vi "134 - Pro - Con (Saved).vi"() -> ()   [LabVIEW 2020]
doc: "Use this template to build a producer/consumer design pattern. Use this template when you need to execute a process, such as data analysis, when a data source, such as a triggered acquisition, produces data at an uneven rate and you need to execute the process when the data becomes available."
uses:
  <vilib>/Utility/error.llb/DialogType.ctl
  <vilib>/DAQmx/read.llb/DAQmx Read (Analog Wfm 1Chan NSamp).vi
  <vilib>/DAQmx/create/channels.llb/DAQmx Create Channel (AI-Voltage-Basic).vi
  <vilib>/DAQmx/configure/timing.llb/DAQmx Timing (Sample Clock).vi
  <vilib>/Analysis/0measdsp.llb/Scaled Time Domain Window (DBL).vi
  <vilib>/DAQmx/miscellaneous.llb/DAQmx Fill In Error Info.vi
  <vilib>/Analysis/NI_AALPro.lvlib
panel:
  in  "Sample per Channel":dbl
  out "dt":dbl
  out "Frequency Peak":dbl format="%0.4f"
  in  "Filename":path=path "C:/Users/Hung/Desktop/TestSave.tdms"
  out "Record Signal":waveform(dbl)(graph)
  in  "Compare":dbl
  out "Filename Out":path
  in  "Saving":bool
  out "RMS":dbl
  out "Numeric 2":i32
  out "Numeric":i32
  out "Waveform Graph":waveform(dbl)(graph)
  out "Data (Consumer Loop)":dbl[](array[numeric])
  in  "stop":bool
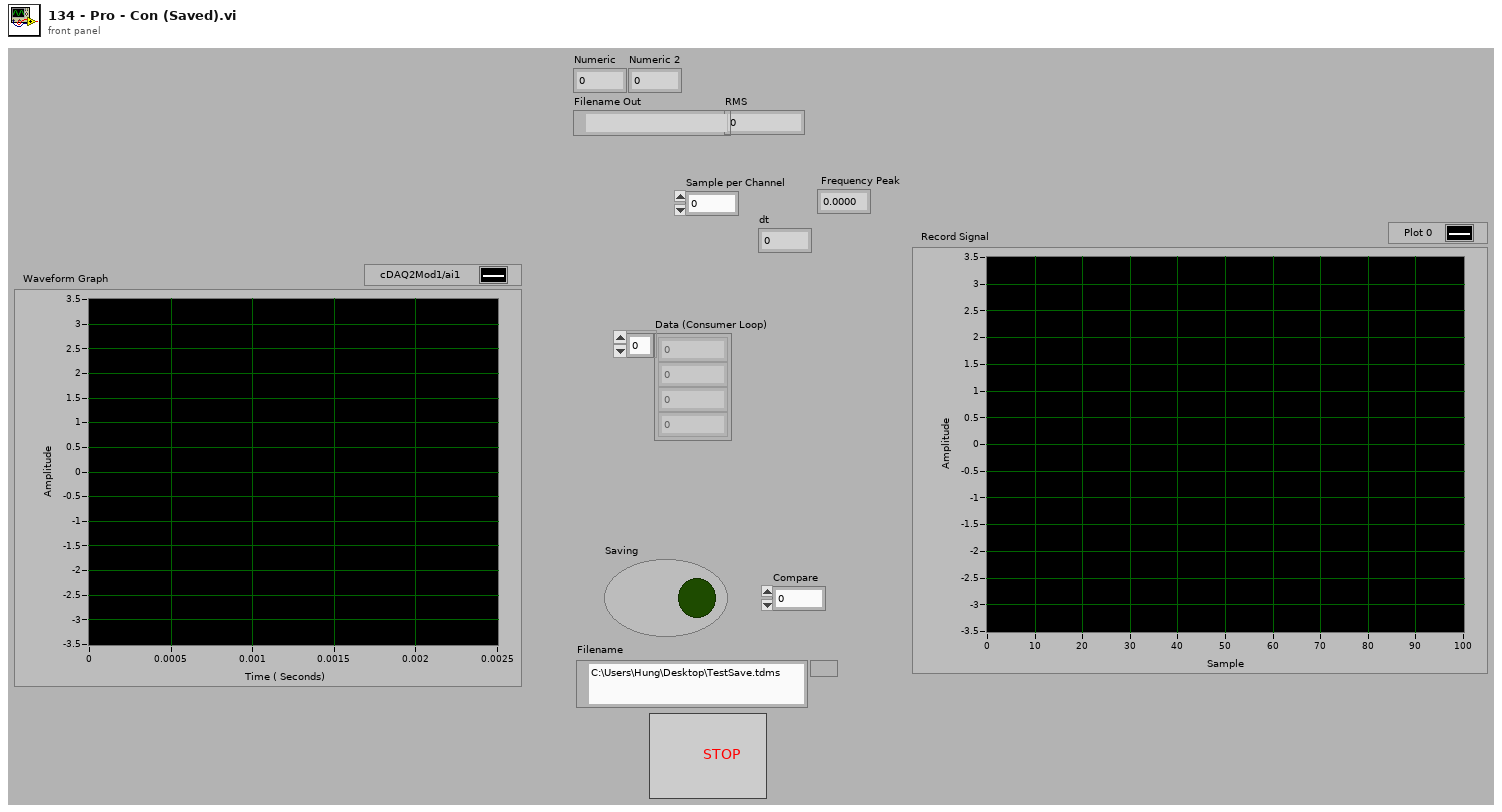
[diagram p1: front panel]
types:
  T1 = typedef "DialogType.ctl" = u16
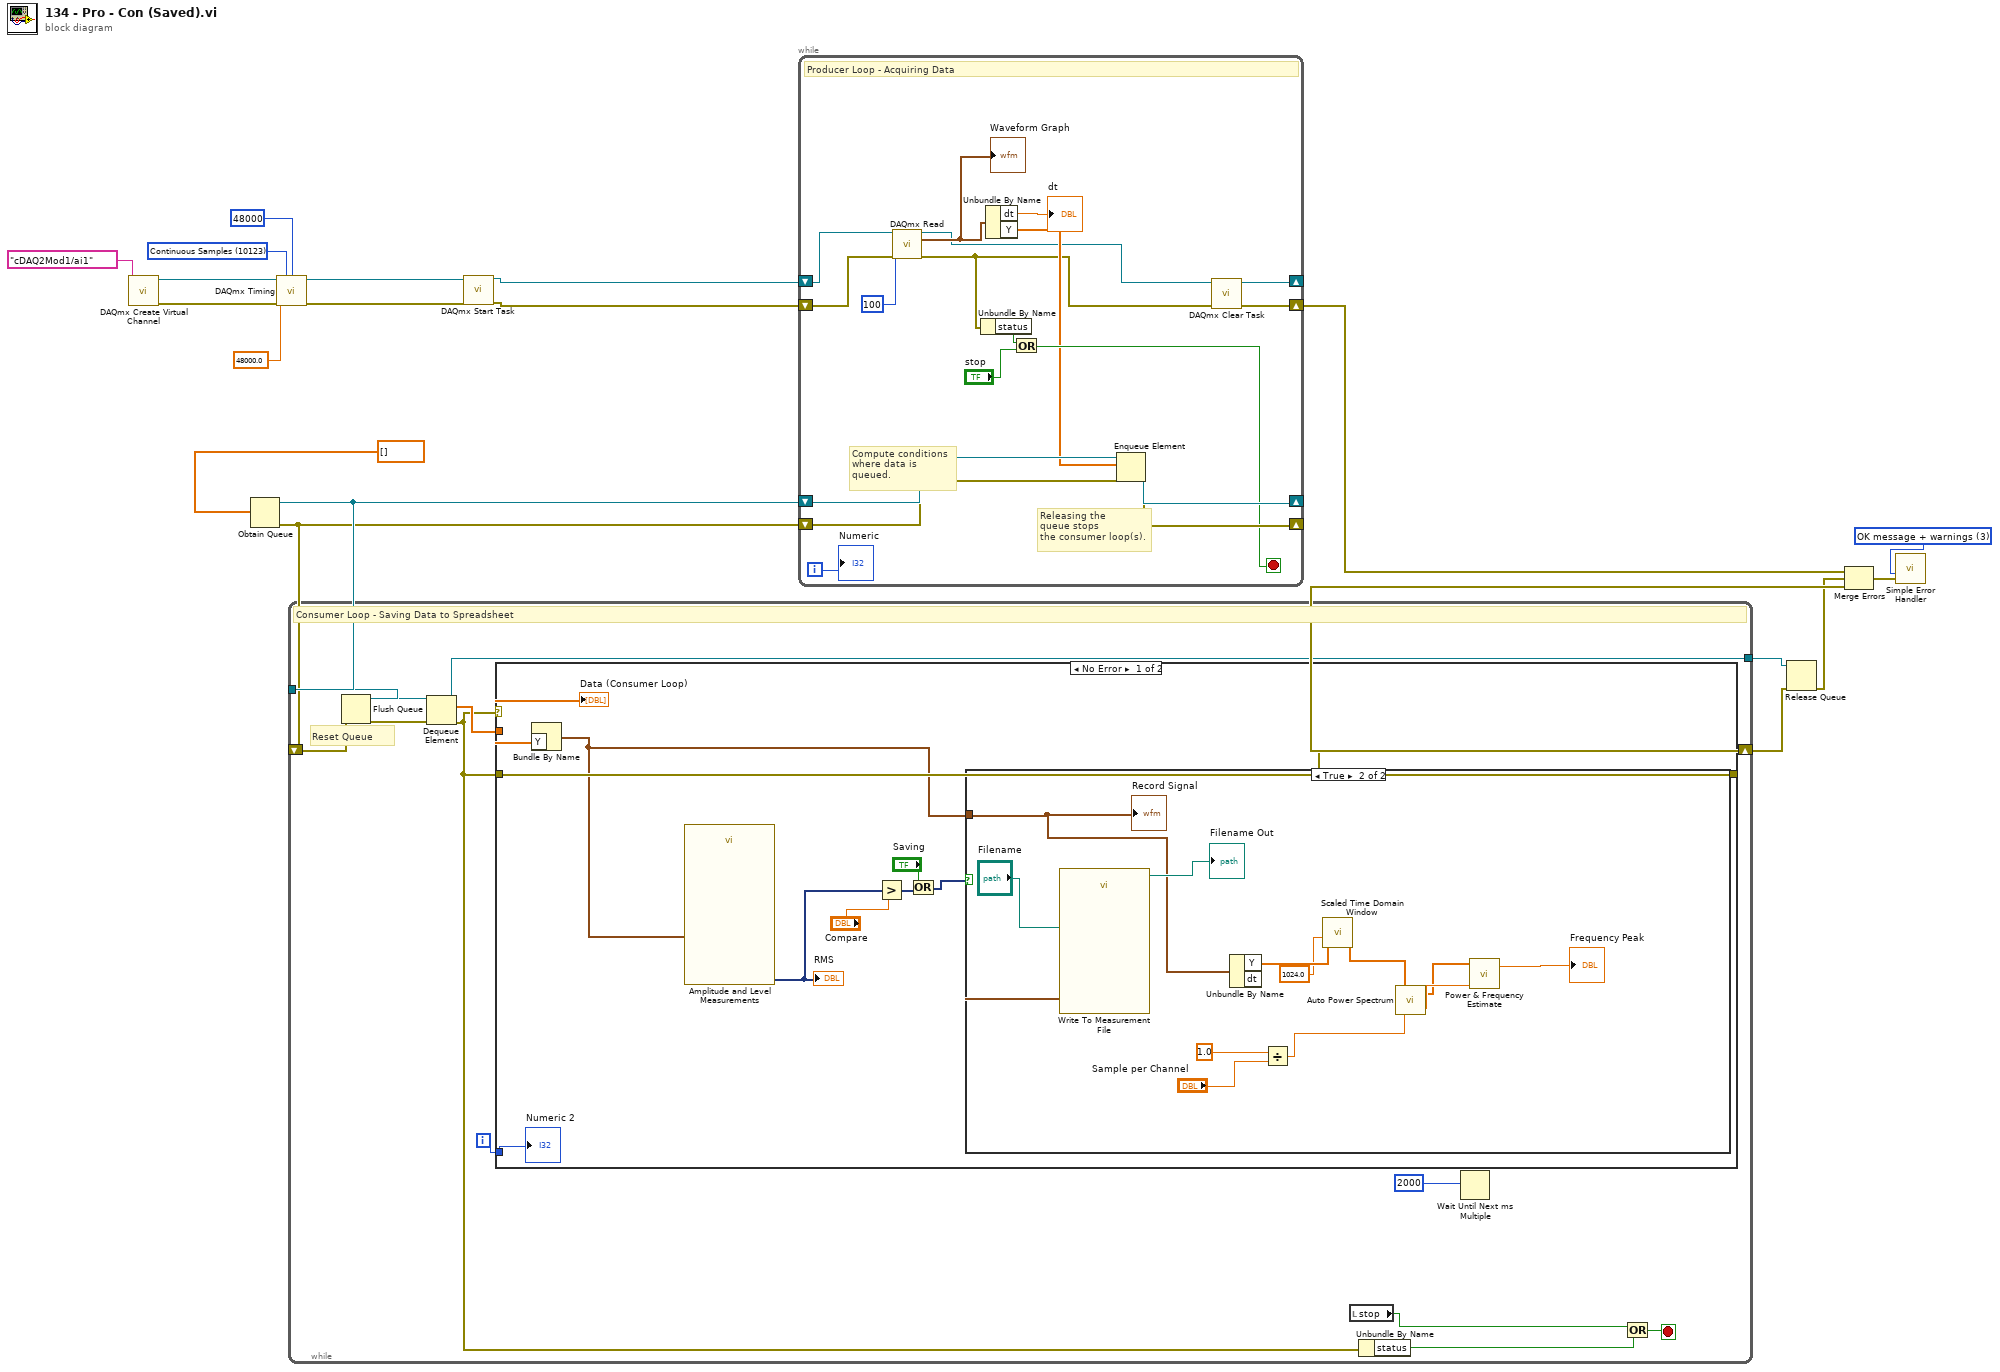
[diagram p0: block diagram]
diagram:
  w13 = 10123 items=["Finite Samples"=10178, "Continuous Samples"=10123, "Hardware Timed Single Point"=12522] ("sample mode")
  w20 = T1 3 items=["no dialog", "OK message", "continue or stop message", "OK message + warnings", "continue/stop + warnings"] ("type of dialog (OK msg:1)")
  n1 = call-poly <vilib>:"DAQmx Create Virtual Channel.vi"("physical channels"=tag "cDAQ2Mod1/ai1") -> ("task out"=w15:refnum<k21>, "error out"=w14:errorcluster)  [unwired: 13 in]
  n2 = Obtain Queue(element data type=dbl[] []) -> (queue out=w21:refnum<queue>, error out=w17:errorcluster)  [unwired: 3 in, 2 out]
  n3 = call-poly <vilib>:"DAQmx Timing.vi"("task/channels in"=w15, "sample mode"=w13, "samples per channel"=48000, "rate"=48000.0, "error in"=w14) -> ("task out"=w11:refnum<k21>, "error out"=w10:errorcluster)  [unwired: 9 in]
  n4 = while {
    tunnel: w21 -> [w25]
    shift-right: [w34] -> w2
    shift-left: w17 -> [w23]
    tunnel: [w26] -> w3
    i -> [w28]
    stop <- w30 stop-if-true
    # "Reset Queue"
    # "Consumer Loop - Saving Data to Spreadsheet"
    n5 = Flush Queue(queue=w25, error in (no error)=w23) -> (queue out=w24:refnum<queue>, error out=w22:errorcluster)  [unwired: 1 out]
    n6 = Dequeue Element(queue=w24, error in (no error)=w22) -> (queue out=w26:refnum<queue>, element=w33:dbl[], error out=w29:errorcluster)  [unwired: 2 out]
    n7 = case shown="No Error" w29 {
      tunnel: w33 -> [w35 _]
      tunnel: [w43 w56] -> w34
      tunnel: w29 -> [w43 w56]
      tunnel: w28 -> [w37 _]
      frame No Error {
        n8 = Bundle By Name("Y"=w35) -> (w36:waveform(dbl))  [unwired: 1 in]
        n9 = call "Amplitude and Level Measurements"("Signals"=w36) -> ("RMS"=w42:dynamicdata)  [unwired: 12 in, 2 out]
        "RMS" <- w42
        n10 = Greater?(x=w42, y="Compare") -> (0:w41:dynamicdata)
        n11 = Or(x="Saving", y=w41) -> (x .or. y?=w39:dynamicdata)
        n12 = case shown="True" w39 {
          tunnel: w36 -> [_ w53]
          frame False {
          }
          frame True {
            n13 = call "Write To Measurement File"("Signals"=w53, "Filename"="Filename") -> ("Filename Out"=→"Filename Out":path)  [unwired: 15 in, 2 out]
            n14 = Unbundle By Name(w53) -> ("Y"=w52:dbl[])  [unwired: 1 out]
            n15 = Divide(x=1.0, y="Sample per Channel") -> (x/y=w44:dbl)
            n16 = call-poly <vilib>:"Scaled Time Domain Window.vi"("window parameter"=1024.0, "X"=w52) -> ("Windowed X"=w51:dbl[])  [unwired: 1 in, 8 out]
            n17 = call <vilib>:"Auto Power Spectrum.vi"("dt"=w44, "Signal (V)"=w51) -> ("df"=w50:dbl, "Power Spectrum (V^2 rms)"=w47:dbl[])
            n18 = call <vilib>:"Power & Frequency Estimate.vi"("df"=w50, "Power Spectrum (V^2 rms)"=w47) -> ("est frequency peak"=→"Frequency Peak":dbl)  [unwired: 3 in, 2 out]
            "Record Signal" <- w53
          }
        }
        "Data (Consumer Loop)" <- w35
        "Numeric 2" <- w37
      }
      frame Error {
      }
    }
    n19 = local read "stop"() -> (w32:bool)
    n20 = Unbundle By Name(w29) -> ("status"=w31:bool)
    n21 = Wait Until Next ms Multiple(millisecond multiple=u32 2000 ("milliseconds to wait")) -> ()  [unwired: 1 out]
    n22 = Or(x=w32, y=w31) -> (x .or. y?=w30:bool)
  }
  n23 = call <vilib>:"DAQmx Start Task.vi"("task/channels in"=w11, "error in"=w10) -> ("task out"=w8:refnum<k21>, "error out"=w7:errorcluster)  [unwired: 12 in]
  n24 = while {
    shift-right: [w69] -> _
    shift-left: w17 -> [w70]
    shift-right: [w71] -> _
    shift-left: w21 -> [w72]
    shift-right: [w61] -> w6
    shift-left: w8 -> [w65]
    shift-right: [w60] -> w5
    shift-left: w7 -> [w64]
    i -> [w59]
    stop <- w66 stop-if-true
    # "Releasing the\nqueue stops\nthe consumer loop(s)."
    # "Compute conditions\nwhere data is\nqueued."
    # "Producer Loop - Acquiring Data"
    n25 = call-poly <vilib>:"DAQmx Read.vi"("task/channels in"=w65, "number of samples per channel"=100, "error in"=w64) -> ("task out"=w61:refnum<k21>, "data"=w62:waveform(dbl), "error out"=w60:errorcluster)  [unwired: 10 in]
    "Waveform Graph" <- w62
    n26 = Unbundle By Name(w60) -> ("status"=w68:bool)
    n27 = Unbundle By Name(w62) -> ("dt"=→"dt":dbl, "Y"=w63:dbl[])
    n28 = Or(x=w68, y="stop") -> (x .or. y?=w66:bool)
    n29 = Enqueue Element(queue=w72, element=w63, error in (no error)=w70) -> (queue out=w71:refnum<queue>, error out=w69:errorcluster)  [unwired: 2 out]
    "Numeric" <- w59
  }
  n30 = call <vilib>:"DAQmx Clear Task.vi"("task in"=w6, "error in"=w5) -> ("error out"=w18:errorcluster)  [unwired: 13 out]
  n31 = Release Queue(queue=w3, error in (no error)=w2) -> (error out=w1:errorcluster)  [unwired: 1 in, 2 out]
  n32 = Merge Errors(w18, w1, w2) -> (w19:errorcluster)
  n33 = call <vilib>:"Simple Error Handler.vi"("type of dialog (OK msg:1)"=w20, "error in (no error)"=w19) -> ()  [unwired: 8 out]
